vi "AMview.vi"() -> ()   [LabVIEW 2014]
uses:
  TypeDefs/Color.ctl
  TypeDefs/SCAN.ctl
  TypeDefs/Poly2DwSlope.ctl
  TypeDefs/Point2DwSlope.ctl
  TypeDefs/CameraEvent.ctl
  TypeDefs/Camera.ctl
  <vilib>/Utility/miscctls.llb/LV3DPointTypeDef.ctl
  <vilib>/Utility/miscctls.llb/LVStringsAndValuesArrayTypeDef_U16.ctl
  TypeDefs/Point3D.ctl
  <vilib>/picture/3D Picture Control/Object/Add Object (no reference).vi
  <vilib>/picture/3D Picture Control/Object/Create Object (name).vi
  <vilib>/xml/Close Reference(Node).vi
  <vilib>/picture/3D Picture Control/NI_3D Picture Control.lvlib
  <vilib>/xml/NI_XML.lvlib
  <resource>/objmgr/DOMUserDefRef.rc
panel:
  out "SCAN":T1
  in  "stop":bool
  in  "Toolbar":T4(tab)
  in  "Load":bool
  in  "Line Width":dbl=1.0
  in  "Color Off":T5={"Alpha"=1.0, "Color"=0} {"Alpha" min=0.0 max=1.0 scale=0.0..1.0}
  in  "Line Color":u32(colorbox)=6618880
  in  "Reset":bool
  in  "Ports":enum16{"One Viewport", "Four Viewports"}(ring)
  in  "Build Plate Color":u32(colorbox)=6618880
  in  "Color On":T5={"Alpha"=1.0, "Color"=0} {"Alpha" min=0.0 max=1.0 scale=0.0..1.0}
  in  "Scale":bool
  in  "Percent":dbl=50.0 min=1.0 max=200.0
  in  "ZT":dbl=1.0
  in  "ZPT":bool
  in  "ZNT":bool
  in  "YT":dbl=1.0
  in  "YPT":bool
  in  "YNT":bool
  in  "XT":dbl=1.0
  in  "XPT":bool
  in  "XNT":bool
  in  "Zcen":dbl
  in  "Ycen":dbl
  in  "Xcen":dbl
  in  "Zmax":dbl
  in  "Zmin":dbl
  in  "Ymax":dbl
  in  "Ymin":dbl
  in  "Xmax":dbl
  in  "Xmin":dbl
  in  "ZR":dbl=90.0
  in  "ZRR":bool
  in  "ZLR":bool
  in  "YR":dbl=90.0
  in  "YRR":bool
  in  "YLR":bool
  in  "XR":dbl=90.0
  in  "XRR":bool
  in  "XLR":bool
  in  "Model Selector":u16(ring) items=["GE_SnapBlock_18x9_Repaired"]
  in  "Model Color":T5={"Alpha"=1.0, "Color"=0} {"Alpha" min=0.0 max=1.0 scale=0.0..1.0}
  in  "Layer Thickness":dbl=1.0
  in  "Beam Size":dbl=1.0
  in  "Build Size":dbl=100.0
  in  "SavePath":bool
  in  "Slice":bool
  in  "Z":dbl
  in  "SaveSCAN":bool
  in  "SaveXML":bool
  in  "GenLayer":bool
  out "XML":string
  # "X-->"
  # "Translation"
  # "Scale/Sym"
  # "Rotation"
  # "Bounds"
  # "Y-->"
  # "Z-->"
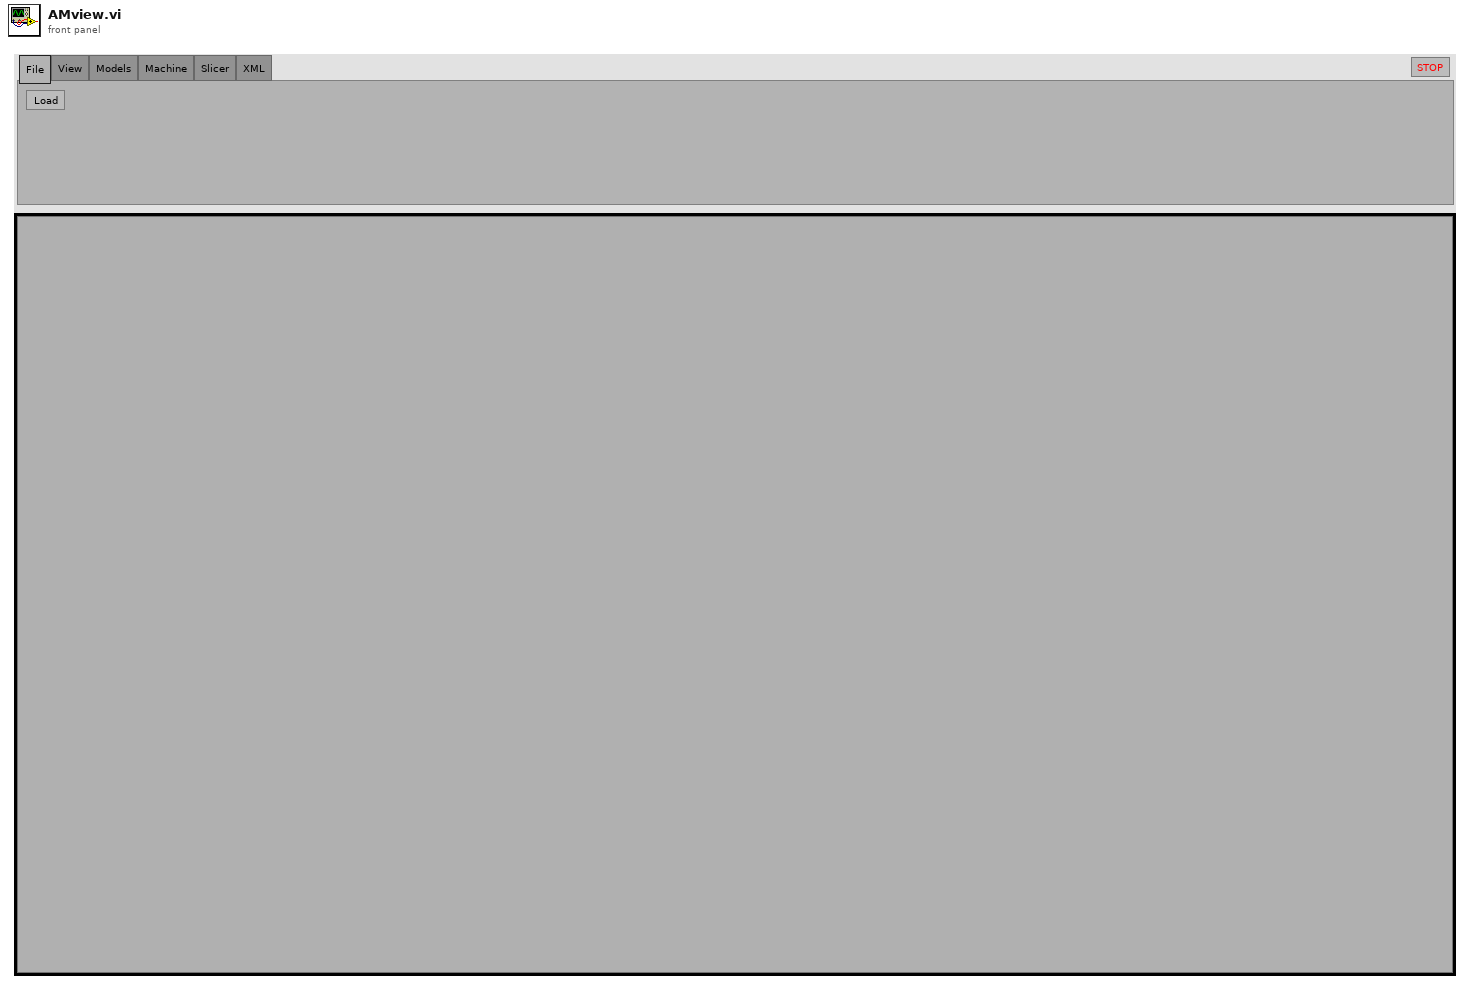
[diagram p1: front panel]
types:
  T1 = typedef "SCAN.ctl" = cluster{"Polys":T2[], "Path":cluster{"VertexArray":T3[], "OnOffAr":enum16{"On", "Off"}[]}}
  T2 = typedef "Poly2DwSlope.ctl" = cluster{"VertexArray":T3[]}
  T3 = typedef "Point2DwSlope.ctl" = cluster{"X":sgl, "Y":sgl, "Slope":dbl}
  T4 = enum32{"File", "View", "Models", "Machine", "Slicer", "XML"}
  T5 = typedef "Color.ctl" = cluster{"Alpha":dbl, "Color":u32}
  T6 = enum16{"Add", "Get", "Scale", "Rotate", "Translate", "Symmetry", "Clear"}
  T7 = enum16{"New", "Find", "FindPattern", "GetTable", "Clear"}
  T8 = typedef "LVStringsAndValuesArrayTypeDef_U16.ctl" = cluster{"String":string, "Value":u16}[]
  T9 = typedef "CameraEvent.ctl" = cluster{"Camera":T10, "Task":enum16{"redraw", "setTo", "setToUpdate"}}
  T10 = typedef "Camera.ctl" = cluster{"Camera Position":T11, "Target":T11, "Up Direction":T11}
  T11 = typedef "LV3DPointTypeDef.ctl" = cluster{"X":sgl, "Y":sgl, "Z":sgl}
  T12 = enum16{"Add", "Get", "Scale", "Rotate", "Translate", "Symmetry"}
  T13 = enum16{"Overall", "Per Primitive", "Per Vertex", "Binding Off"}
  T14 = enum16{"Points", "Lines", "Line Strip", "Line Loop", "Triangles", "Triangle Strip", "Triangle Fan", "Quads", "Quad Strip", "Polygon"}
  T15 = cluster{"Axis":enum16{"X", "Y", "Z"}, "Angle":sgl}
  T16 = typedef "Point3D.ctl" = cluster{"X":sgl, "Y":sgl, "Z":sgl}
  T17 = typedef "TriangleFace.ctl" = cluster{"Normal":T16, "Vertex1":T16, "Vertex2":T16, "Vertex3":T16}
  T18 = typedef "Line2D.ctl" = cluster{"Vertex1":T3, "Vertex2":T3, "Slope":dbl}
  T19 = cluster{"VertexArray":T3[], "OnOffAr":enum16{"On", "Off"}[]}
  T20 = cluster{"Polys":T2[], "Path":cluster{"VertexArray":T3[], "OnOffAr":enum16{"On", "Off"}[]}}
  T21 = cluster{"VertexArray":T3[], enum16{"On", "Off"}[]}
  T22 = cluster{"VertexArray":T3[], "OnOffAr":enum16{"On", "Off"}[]}[]
  T23 = typedef "XYonOffArray.ctl" = cluster{"X":dbl, "Y":dbl, "OnOff":bool}[]
  T24 = typedef "LVRGBAColorTypeDef.ctl" = cluster{"Red":sgl, "Green":sgl, "Blue":sgl, "Alpha":sgl}
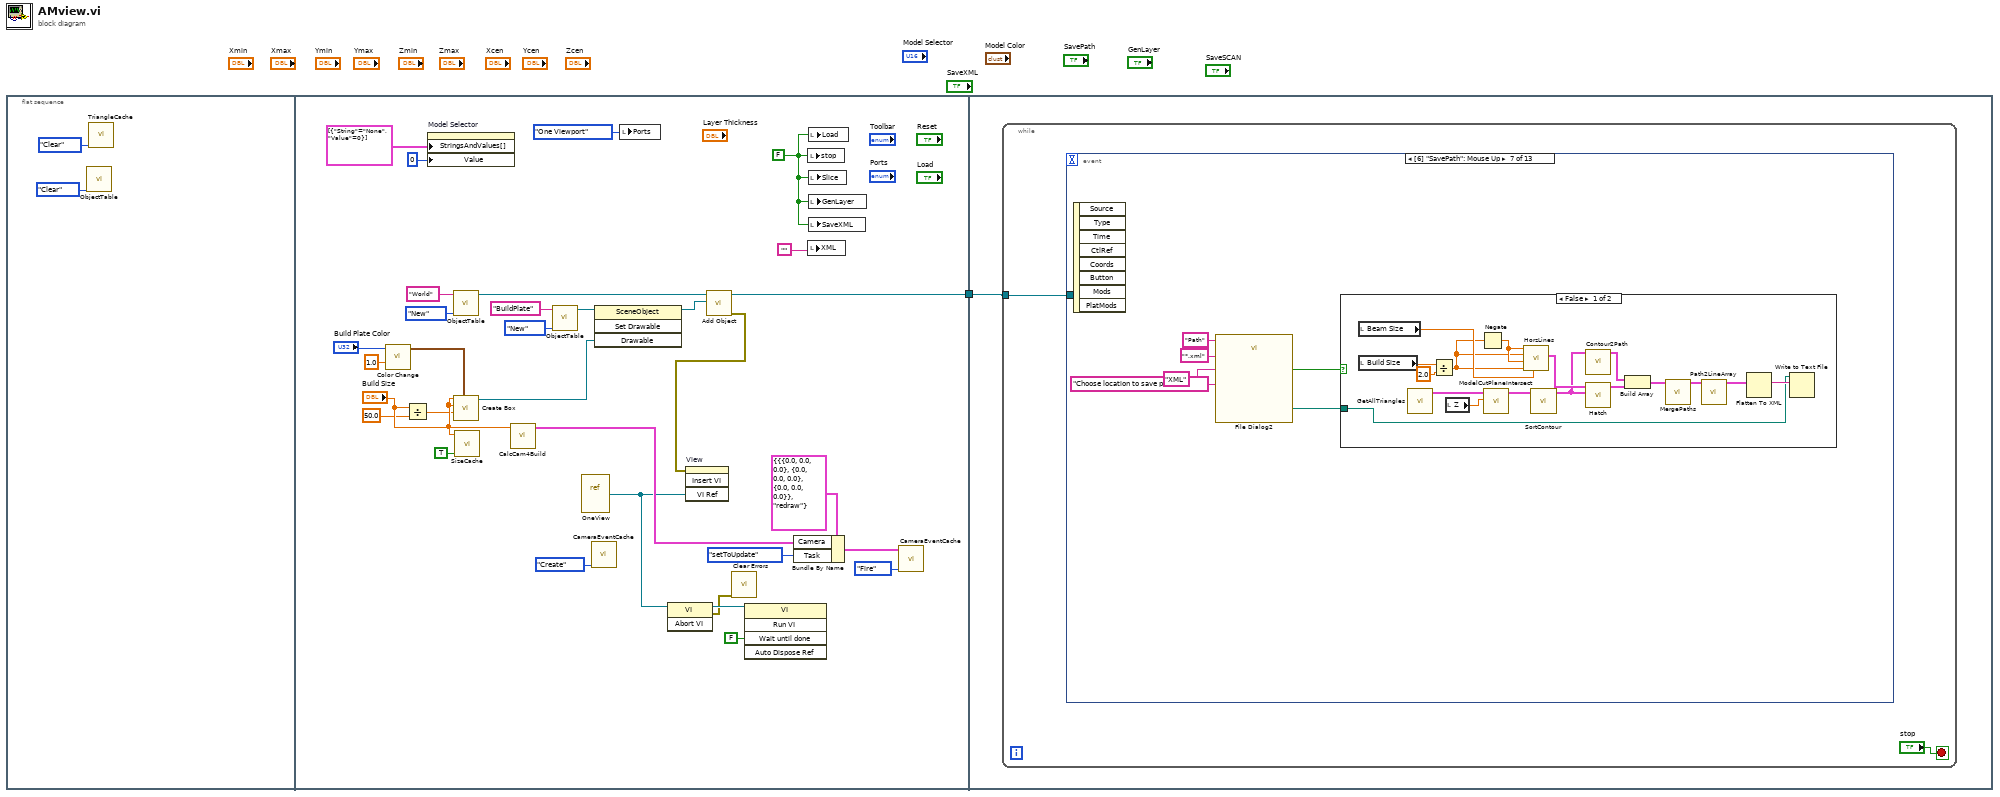
[diagram p0: block diagram]
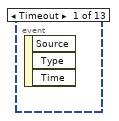
[diagram p2: hidden frame]
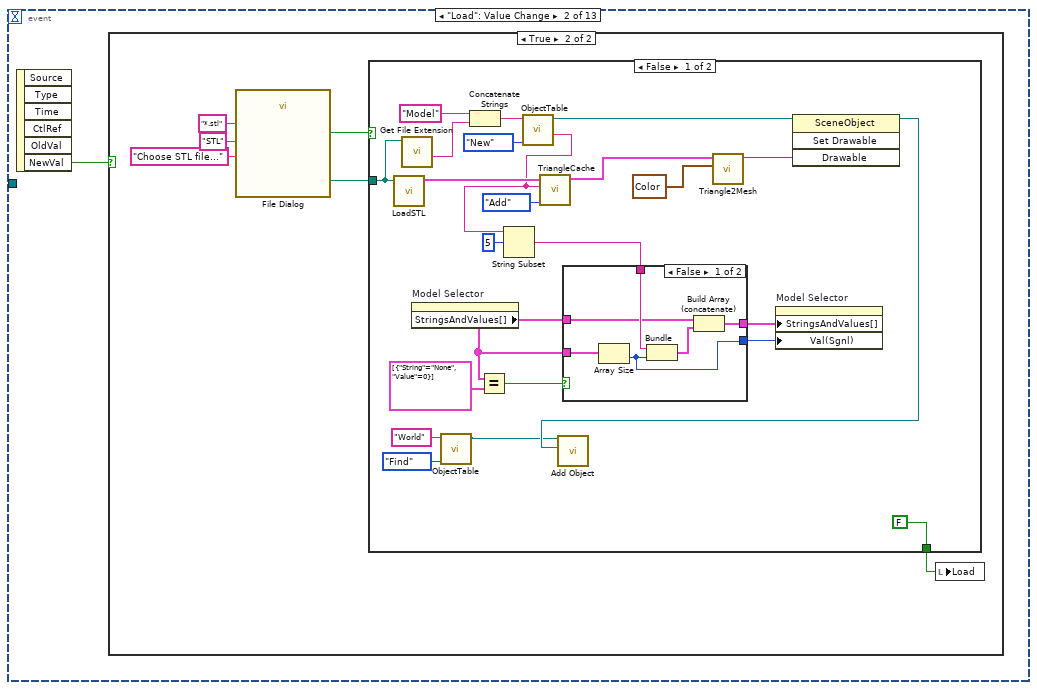
[diagram p3: hidden frame]
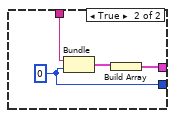
[diagram p5: hidden frame]
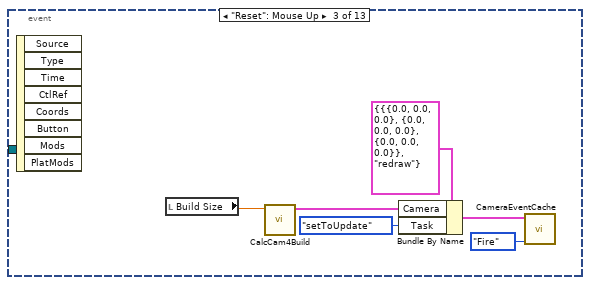
[diagram p7: hidden frame]
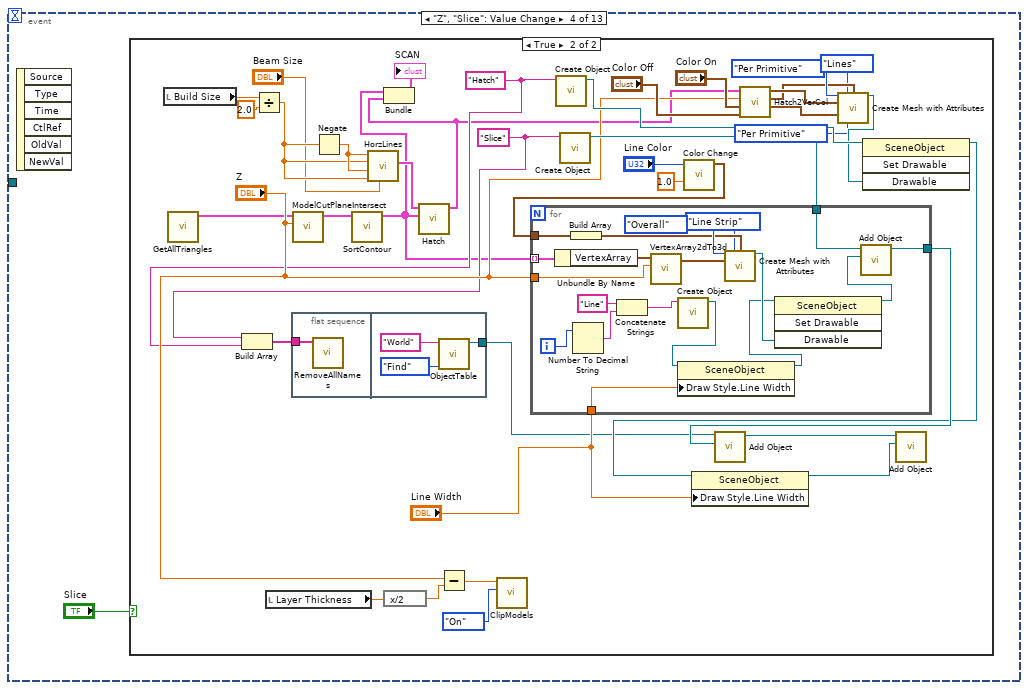
[diagram p8: hidden frame]
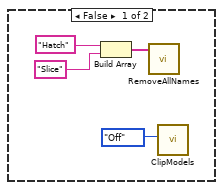
[diagram p9: hidden frame]
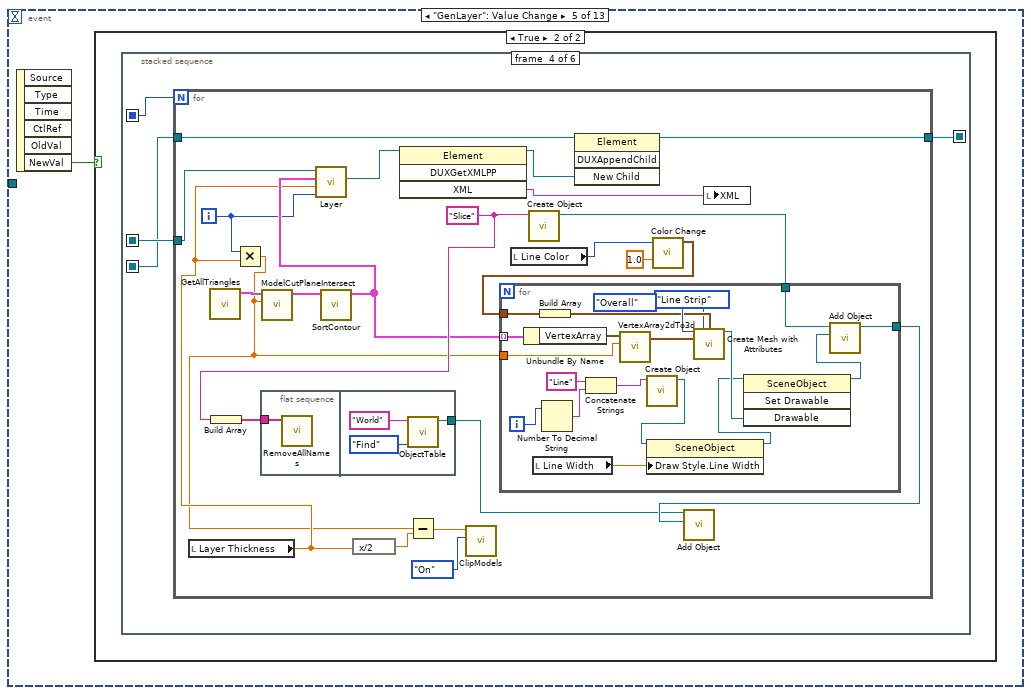
[diagram p10: hidden frame]
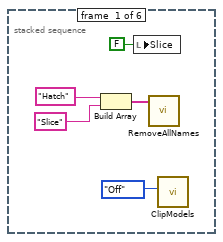
[diagram p12: hidden frame]
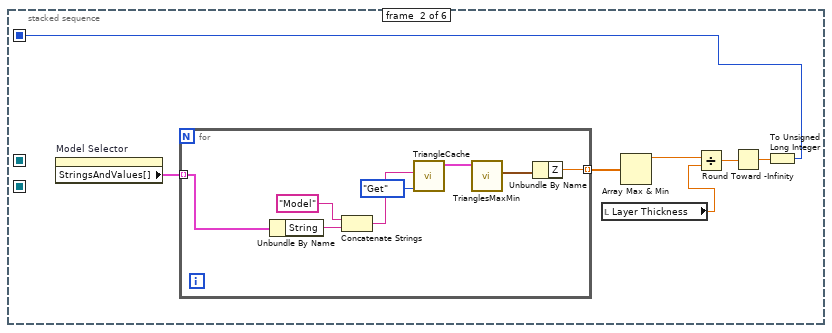
[diagram p13: hidden frame]
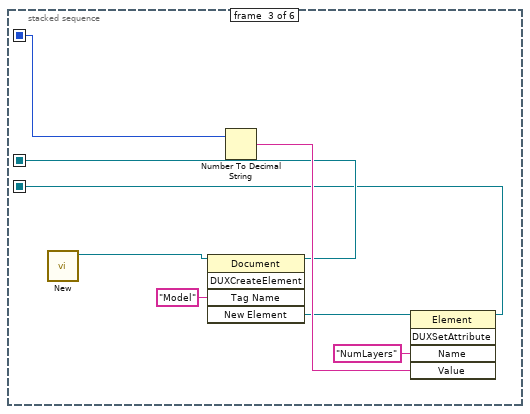
[diagram p14: hidden frame]
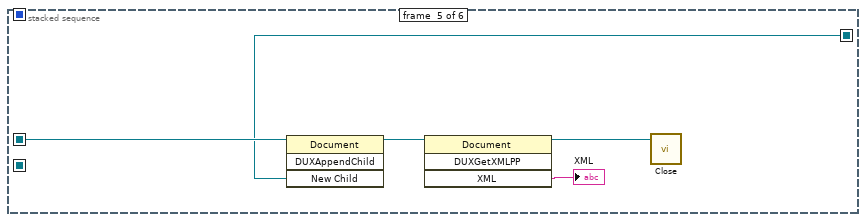
[diagram p15: hidden frame]
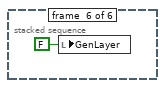
[diagram p16: hidden frame]
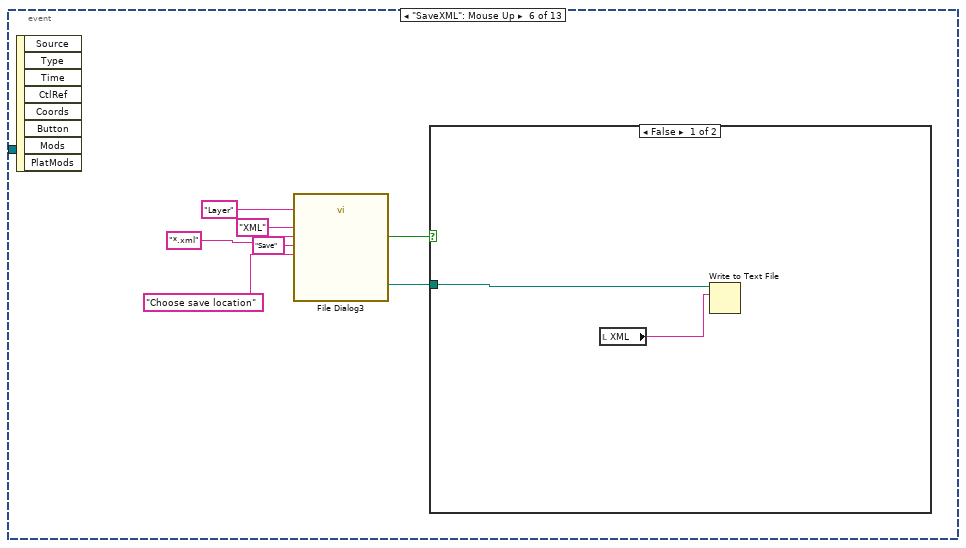
[diagram p17: hidden frame]
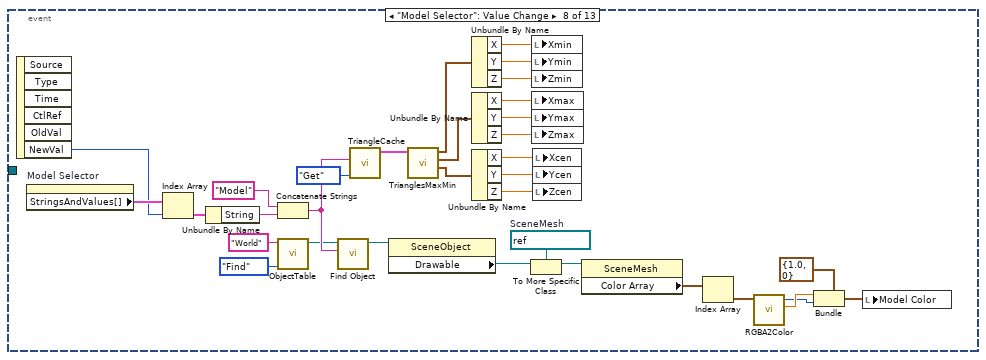
[diagram p20: hidden frame]
diagram:
  n1 = flat-sequence {
    tunnel: [w13] -> w1
    tunnel: w1 -> [w36]
    frame #0 {
      n2 = call "ObjectTable.vi"("ObjectStoreSelector"=T7."Clear") -> ()  [unwired: 6 in, 5 out]
      n3 = call "TriangleCache.vi"("TriangleOperations"=T6."Clear") -> ()  [unwired: 10 in, 1 out]
    }
    frame #1 {
      w5 = FALSE ("stop")
      n4 = call <vilib>:"Color Change.vi"("Alpha"=1.0, "Color"="Build Plate Color") -> ("RGBA"=w17:cluster{"R":sgl, "G":sgl, "B":sgl, "A":sgl})  [unwired: 9 in]
      n5 = Divide(x="Build Size", y=50.0) -> (x/y=w15:dbl)
      n6 = property on="Model Selector" class="Ring (strict)"("StringsAndValues[]"=T8 [{"String"="None", "Value"=0}] ("Strings And Values []"), "Value"=0) -> ()  [unwired: 2 in, 2 out]
      n7 = call "ObjectTable.vi"("ObjectStoreSelector"=enum16{"New", "Find", "FindPattern", "GetTable"}."New", "Name"="World") -> ("ObjectRef"=w31:refnum<vi>)  [unwired: 5 in, 4 out]
      n8 = call <vilib>:"Create Box.vi"("Color"=w17, "Length Z"=w15, "Length Y"="Build Size", "Length X"="Build Size") -> ("New Box Refnum"=w19:refnum<vi>)  [unwired: 6 in, 1 out]
      n9 = call "SizeCache.vi"("Set"=TRUE, "SizeIn"="Build Size") -> ()  [unwired: 9 in, 1 out]
      n10 = call "CalcCam4Build.vi"("BuildSize"="Build Size") -> ("CamOut"=w25:T10)  [unwired: 10 in]
      n11 = call "ObjectTable.vi"("ObjectStoreSelector"=enum16{"New", "Find", "FindPattern", "GetTable"}."New", "Name"="BuildPlate") -> ("ObjectRef"=w33:refnum<vi>)  [unwired: 5 in, 4 out]
      n12 = vi-ref "OneView.vi"() -> (w9:refnum<vi>)
      n13 = call "CameraEventCache.vi"("Operation"=enum16{"Create", "GetRef", "Fire"}."Create") -> ()  [unwired: 10 in, 1 out]
      n14 = invoke class="SceneObject" method="Set Drawable"(reference=w33, "Drawable"=w19) -> (reference out=w20:refnum<vi>)  [unwired: 2 in, 3 out]
      n15 = local write "Ports"(enum16{"One Viewport", "Four Viewports"}."One Viewport" ("Ports")) -> ()
      n16 = invoke class="VI" method="Abort VI"(reference=w9) -> (reference out=w10:refnum<vi>, error out=w6:errorcluster)  [unwired: 2 in, 1 out]
      n17 = call-poly <vilib>:"Add Object.vi"("New Object In"=w20, "Scene Object In"=w31) -> ("error out"=w35:errorcluster, "Scene Object Out"=w13:refnum<vi>)  [unwired: 8 in]
      n18 = invoke on="View" class="SubPanel" method="Insert VI"(error in=w35, "VI Ref"=w9) -> ()  [unwired: 2 in, 4 out]
      n19 = call <vilib>:"Clear Errors.vi"("error in (no error)"=w6) -> ()  [unwired: 5 in, 2 out]
      n20 = invoke class="VI" method="Run VI"(reference=w10, "Wait until done"=FALSE ("Wait Until Done")) -> ()  [unwired: 3 in, 5 out]
      n21 = Bundle By Name(cluster=T9 {"Camera"={"Camera Position"={"X"=0.0, "Y"=0.0, "Z"=0.0}, "Target"={"X"=0.0, "Y"=0.0, "Z"=0.0}, "Up Direction"={"X"=0.0, "Y"=0.0, "Z"=0.0}}, "Task"=enum."redraw"} ("CameraEvent"), "Camera"=w25, "Task"=enum16{"redraw", "setTo", "setToUpdate"}."setToUpdate") -> (w24:T9)
      n22 = local write "stop"(w5) -> ()
      n23 = local write "XML"("") -> ()
      n24 = local write "Load"(w5) -> ()
      n25 = local write "Slice"(w5) -> ()
      n26 = local write "GenLayer"(w5) -> ()
      n27 = local write "SaveXML"(w5) -> ()
      n28 = call "CameraEventCache.vi"("Operation"=enum16{"Create", "GetRef", "Fire"}."Fire", "CameraEvent"=w24) -> ()  [unwired: 9 in, 1 out]
    }
    frame #2 {
      n29 = while {
        tunnel: w36 -> [w37]
        stop <- "stop" stop-if-true
        n30 = event shown="[6] \"SavePath\": Mouse Up" {
          selector: _ -> [_ _ _ _ _ _ _ _ _ _ _ _ _]
          dyn-events: _ -> [_ _ _ _ _ _ _ _ _ _ _ _ _]
          timeout: _ -> [_ _ _ _ _ _ _ _ _ _ _ _ _]
          tunnel: w37 -> [_ _ _ _ _ _ _ _ _ _ _ _ _]
          event Timeout {
            n31 = event-data() -> ()  [unwired: 1 in, 3 out]
          }
          event "Load": Value Change {
            n32 = event-data() -> ("NewVal"=w39:bool)  [unwired: 1 in, 5 out]
            n33 = case shown="True" w39 {
              frame False {
              }
              frame True {
                n34 = call "File Dialog"("prompt"="Choose STL file...", "pattern (all files)"="*.stl", "pattern label"="STL") -> ("selected path"=w41:path, "cancelled"=w42:bool)  [unwired: 9 in, 2 out]
                n35 = case shown="False" w42 {
                  tunnel: w41 -> [w54 _]
                  tunnel: [FALSE _] -> w40
                  frame False {
                    n36 = call "LoadSTL.vi"("STL Path"=w54) -> ("Triangles"=w59:T17[])  [unwired: 8 in, 2 out]
                    n37 = call <vilib>:"Get File Extension.vi"("file"=w54) -> ("filename without extension"=w53:string)  [unwired: 7 in, 3 out]
                    n38 = property on="Model Selector" class="Ring (strict)"() -> ("StringsAndValues[]"=w48:T8)  [unwired: 2 in, 2 out]
                    n39 = call "ObjectTable.vi"("ObjectStoreSelector"=enum16{"New", "Find", "FindPattern", "GetTable"}."Find", "Name"="World") -> ("ObjectRef"=w63:refnum<vi>)  [unwired: 5 in, 4 out]
                    n40 = Concatenate Strings("Model" ("Name"), w53) -> (w66:string)
                    n41 = Equal?(x=w48, y=T8 [{"String"="None", "Value"=0}] ("Strings And Values []")) -> (x = y?=w47:bool)
                    n42 = call "ObjectTable.vi"("ObjectStoreSelector"=enum16{"New", "Find", "FindPattern", "GetTable"}."New", "Name"=w66) -> ("UniqueName"=w51:string, "ObjectRef"=w64:refnum<vi>)  [unwired: 5 in, 3 out]
                    n43 = String Subset(string=w51, offset (0)=5) -> (substring=w52:string)  [unwired: 1 in]
                    n44 = call "TriangleCache.vi"("TriangleOperations"=T12."Add", "ModelName"=w51, "TrianglesIn"=w59) -> ("TrianglesOut"=w58:T17[])  [unwired: 8 in]
                    n45 = case shown="False" w47 {
                      tunnel: [w74 w77] -> w56
                      tunnel: [w73 w76] -> w55
                      tunnel: w52 -> [w72 w79]
                      tunnel: w48 -> [w71 _]
                      tunnel: w48 -> [w70 _]
                      frame False {
                        n46 = Array Size(array=w70) -> (size(s)=w73:i32)
                        n47 = Bundle("UniqueName"=w72, w73) -> (w75:cluster{"UniqueName":string, i32})  [unwired: 1 in]
                        n48 = Build Array (concatenate)(w71, w75) -> (w74:cluster{"UniqueName":string, "Value":i32}[])
                      }
                      frame True {
                        w76 = 0
                        n49 = Bundle("UniqueName"=w79, w76) -> (w78:cluster{"UniqueName":string, i32})  [unwired: 1 in]
                        n50 = Build Array(w78) -> (w77:cluster{"UniqueName":string, i32}[])
                      }
                    }
                    n51 = call "Triangle2Mesh.vi"("Color"=T5 {"Alpha"=1.0, "Color"=16711680}, "Triangles"=w58) -> ("Refnum"=w60:refnum<vi>)  [unwired: 9 in]
                    n52 = property on="Model Selector" class="Ring (strict)"("StringsAndValues[]"=w56, "Val(Sgnl)"=w55) -> ()  [unwired: 2 in, 2 out]
                    n53 = invoke class="SceneObject" method="Set Drawable"(reference=w64, "Drawable"=w60) -> (reference out=w69:refnum<vi>)  [unwired: 2 in, 3 out]
                    n54 = call-poly <vilib>:"Add Object.vi"("New Object In"=w69, "Scene Object In"=w63) -> ()  [unwired: 8 in, 2 out]
                  }
                  frame True {
                  }
                }
                n55 = local write "Load"(w40) -> ()
              }
            }
          }
          event "Reset": Mouse Up {
            n56 = event-data() -> ()  [unwired: 1 in, 8 out]
            n57 = local read "Build Size"() -> (w82:dbl)
            n58 = call "CalcCam4Build.vi"("BuildSize"=w82) -> ("CamOut"=w83:T10)  [unwired: 10 in]
            n59 = Bundle By Name(cluster=T9 {"Camera"={"Camera Position"={"X"=0.0, "Y"=0.0, "Z"=0.0}, "Target"={"X"=0.0, "Y"=0.0, "Z"=0.0}, "Up Direction"={"X"=0.0, "Y"=0.0, "Z"=0.0}}, "Task"=enum."redraw"} ("CameraEvent"), "Camera"=w83, "Task"=enum16{"redraw", "setTo", "setToUpdate"}."setToUpdate") -> (w81:T9)
            n60 = call "CameraEventCache.vi"("Operation"=enum16{"Create", "GetRef", "Fire"}."Fire", "CameraEvent"=w81) -> ()  [unwired: 9 in, 1 out]
          }
          event "Z", "Slice": Value Change {
            n61 = event-data() -> ()  [unwired: 1 in, 6 out]
            n62 = case shown="True" "Slice" {
              frame False {
                n63 = Build Array("Hatch", "Slice") -> (w89:string[])
                n64 = call "RemoveAllNames.vi"("Names"=w89) -> ()  [unwired: 11 in]
                n65 = call "ClipModels.vi"("Clip Plane State"=enum16{"Inherit Value", "Off", "On"}."Off") -> ()  [unwired: 11 in]
              }
              frame True {
                w96 = "Hatch" ("Name")
                w97 = "Slice" ("Name")
                n66 = local read "Build Size"() -> (w127:dbl)
                n67 = call "GetAllTriangles.vi"() -> ("AllTriangles"=w100:T17[])  [unwired: 11 in]
                n68 = Build Array(w97, w96) -> (w95:string[])
                n69 = Divide(x=w127, y=2.0) -> (x/y=w124:dbl)
                n70 = local read "Layer Thickness"() -> (w102:dbl)
                n71 = flat-sequence {
                  tunnel: w95 -> [w130]
                  tunnel: [w131] -> w94
                  frame #0 {
                    n72 = call "RemoveAllNames.vi"("Names"=w130) -> ()  [unwired: 11 in]
                  }
                  frame #1 {
                    n73 = call "ObjectTable.vi"("ObjectStoreSelector"=T7."Find", "Name"="World") -> ("ObjectRef"=w131:refnum<vi>)  [unwired: 5 in, 4 out]
                  }
                }
                n74 = call "ModelCutPlaneIntersect.vi"("CuttingZ"="Z", "Triangles"=w100) -> ("LineArray"=w129:T18[])  [unwired: 8 in, 1 out]
                n75 = Negate(x=w124) -> (-x=w125:dbl)
                n76 = call "SortContour.vi"("LineArray"=w129) -> ("Polys"=w93:T2[])  [unwired: 10 in]
                n77 = call "HorzLines.vi"("Spacing"="Beam Size", "yMax"=w124, "yMin"=w125, "xMax"=w124, "xMin"=w125) -> ("Poly2D"=w128:T2)  [unwired: 5 in, 1 out]
                n78 = expression code="x/2"(w102) -> (w101:dbl)
                n79 = call "Hatch.vi"("Polys"=w93, "Hatch"=w128) -> ("Path"=w92:T19)  [unwired: 9 in]
                n80 = Bundle("Polys"=w93, "Path"=w92) -> (→"SCAN":T20)  [unwired: 1 in]
                n81 = Subtract(x="Z", y=w101) -> (x-y=w99:dbl)
                n82 = call "ClipModels.vi"("Clip Plane State"=enum16{"Inherit Value", "Off", "On"}."On", "Z"=w99) -> ()  [unwired: 10 in]
                n83 = call-poly <vilib>:"Create Object.vi"("Name"=w96) -> ("Scene:New Object"=w112:refnum<vi>)  [unwired: 9 in, 1 out]
                n84 = call-poly <vilib>:"Create Object.vi"("Name"=w97) -> ("Scene:New Object"=w121:refnum<vi>)  [unwired: 9 in, 1 out]
                n85 = call <vilib>:"Color Change.vi"("Alpha"=1.0, "Color"="Line Color") -> ("RGBA"=w122:cluster{"R":sgl, "G":sgl, "B":sgl, "A":sgl})  [unwired: 9 in]
                n86 = for {
                  tunnel: w93 -> [w151] mode=indexing
                  tunnel: "Z" -> [w149]
                  tunnel: w122 -> [w147]
                  tunnel: w121 -> [w140]
                  tunnel: [w139] -> w120
                  tunnel: "Line Width" -> [w134]
                  i -> [w143]
                  n87 = Unbundle By Name(w151) -> ("VertexArray"=w150:T3[])
                  n88 = Build Array(w147) -> (w146:cluster{"R":sgl, "G":sgl, "B":sgl, "A":sgl}[])
                  n89 = Number To Decimal String(number=w143) -> (decimal integer string=w142:string)  [unwired: 1 in]
                  n90 = Concatenate Strings("Line" ("string"), w142) -> (w141:string)
                  n91 = call "VertexArray2dTo3d.vi"("Z"=w149, "VertexArray2D"=w150) -> ("VertexArray3D"=w148:T16[])  [unwired: 9 in]
                  n92 = call-poly <vilib>:"Create Object.vi"("Name"=w141) -> ("Scene:New Object"=w136:refnum<vi>)  [unwired: 9 in, 1 out]
                  n93 = property class="SceneObject"(reference=w136, "Draw Style.Line Width"=w134) -> (reference out=w135:refnum<vi>)  [unwired: 1 in, 1 out]
                  n94 = call <vilib>:"Create Mesh with Attributes.vi"("Draw Mode"=T14."Line Strip", "Color Binding Mode"=T13."Overall", "Color Array"=w146, "Vertex Array"=w148) -> ("New Mesh Refnum"=w138:refnum<vi>)  [unwired: 10 in, 1 out]
                  n95 = invoke class="SceneObject" method="Set Drawable"(reference=w135, "Drawable"=w138) -> (reference out=w137:refnum<vi>)  [unwired: 2 in, 3 out]
                  n96 = call-poly <vilib>:"Add Object.vi"("New Object In"=w137, "Scene Object In"=w140) -> ("Scene Object Out"=w139:refnum<vi>)  [unwired: 8 in, 1 out]
                }
                n97 = call-poly <vilib>:"Add Object.vi"("New Object In"=w120, "Scene Object In"=w94) -> ("Scene Object Out"=w110:refnum<vi>)  [unwired: 8 in, 1 out]
                n98 = call "Hatch2VerCol.vi"("Color Off"="Color Off", "Color On"="Color On", "Z"="Z", "Path"=w92) -> ("Normals"=w105:T16[], "Colors"=w114:cluster{"R":sgl, "G":sgl, "B":sgl, "A":sgl}[], "VertexArray3d"=w115:T16[])  [unwired: 5 in]
                n99 = call <vilib>:"Create Mesh with Attributes.vi"("Draw Mode"=T14."Lines", "Color Binding Mode"=T13."Per Primitive", "Color Array"=w114, "Vertex Array"=w115, "Normal Array"=w105, "Normal Binding Mode"=T13."Per Primitive") -> ("New Mesh Refnum"=w111:refnum<vi>)  [unwired: 8 in, 1 out]
                n100 = invoke class="SceneObject" method="Set Drawable"(reference=w112, "Drawable"=w111) -> (reference out=w108:refnum<vi>)  [unwired: 2 in, 3 out]
                n101 = property class="SceneObject"(reference=w108, "Draw Style.Line Width"="Line Width") -> (reference out=w106:refnum<vi>)  [unwired: 1 in, 1 out]
                n102 = call-poly <vilib>:"Add Object.vi"("New Object In"=w106, "Scene Object In"=w110) -> ()  [unwired: 8 in, 2 out]
              }
            }
          }
          event "GenLayer": Value Change {
            n103 = event-data() -> ("NewVal"=w153:bool)  [unwired: 1 in, 5 out]
            n104 = case shown="True" w153 {
              frame False {
              }
              frame True {
                n105 = stacked-sequence {
                  seq-local: [_ w159 _ _ _ _] -> [_ _ w176 w185 _ _]
                  seq-local: [_ _ w175 _ _ _] -> [_ _ _ w184 w236 _]
                  seq-local: [_ _ w174 _ _ _] -> [_ _ _ w183 _ _]
                  seq-local: [_ _ _ w182 _ _] -> [_ _ _ _ w235 _]
                  frame #0 {
                    n106 = Build Array("Hatch", "Slice") -> (w156:string[])
                    n107 = local write "Slice"(FALSE ("Slice")) -> ()
                    n108 = call "RemoveAllNames.vi"("Names"=w156) -> ()  [unwired: 11 in]
                    n109 = call "ClipModels.vi"("Clip Plane State"=enum16{"Inherit Value", "Off", "On"}."Off") -> ()  [unwired: 11 in]
                  }
                  frame #1 {
                    n110 = property on="Model Selector" class="Ring (strict)"() -> ("StringsAndValues[]"=w165:T8)  [unwired: 2 in, 2 out]
                    n111 = for {
                      tunnel: w165 -> [w168] mode=indexing
                      tunnel: [w166] -> w164 mode=indexing
                      n112 = Unbundle By Name(w168) -> ("String"=w173:string)
                      n113 = Concatenate Strings("Model" ("string"), w173) -> (w169:string)
                      n114 = call "TriangleCache.vi"("TriangleOperations"=T6."Get", "ModelName"=w169) -> ("TrianglesOut"=w170:T17[])  [unwired: 9 in]
                      n115 = call "TrianglesMaxMin.vi"("Triangles"=w170) -> ("MaxDims"=w167:T16)  [unwired: 8 in, 2 out]
                      n116 = Unbundle By Name(w167) -> ("Z"=w166:sgl)
                    }
                    n117 = local read "Layer Thickness"() -> (w162:dbl)
                    n118 = Array Max & Min(array=w164) -> (max value=w163:sgl)  [unwired: 3 out]
                    n119 = Divide(x=w163, y=w162) -> (x/y=w161:dbl)
                    n120 = Round Toward -Infinity(1:w161) -> (0:w160:dbl)
                    n121 = To Unsigned Long Integer(number=w160) -> (unsigned 32bit integer=w159:u32)
                  }
                  frame #2 {
                    n122 = call <vilib>:"New.vi"() -> ("DOM document out"=w178:refnum<k20>)  [unwired: 8 in, 1 out]
                    n123 = invoke class="Document" method="DUXCreateElement"(reference=w178, "Tag Name"="Model") -> (reference out=w175:refnum<k20>, "New Element"=w177:refnum<k20>)  [unwired: 3 in, 3 out]
                    n124 = Number To Decimal String(number=w176) -> (decimal integer string=w179:string)  [unwired: 1 in]
                    n125 = invoke class="Element" method="DUXSetAttribute"(reference=w177, "Name"="NumLayers", "Value"=w179) -> (reference out=w174:refnum<k20>)  [unwired: 2 in, 4 out]
                  }
                  frame #3 {
                    n126 = for {
                      N: w185 -> [_]
                      tunnel: w184 -> [w195]
                      tunnel: w183 -> [w193]
                      tunnel: [w192] -> w182
                      i -> [w191]
                      w198 = "Slice" ("Name")
                      n127 = local read "Layer Thickness"() -> (w190:dbl)
                      n128 = call "GetAllTriangles.vi"() -> ("AllTriangles"=w201:T17[])  [unwired: 11 in]
                      n129 = Build Array(w198) -> (w197:string[])
                      n130 = Multiply(x=w191, y=w190) -> (x*y=w189:dbl)
                      n131 = flat-sequence {
                        tunnel: w197 -> [w209]
                        tunnel: [w210] -> w196
                        frame #0 {
                          n132 = call "RemoveAllNames.vi"("Names"=w209) -> ()  [unwired: 11 in]
                        }
                        frame #1 {
                          n133 = call "ObjectTable.vi"("ObjectStoreSelector"=T7."Find", "Name"="World") -> ("ObjectRef"=w210:refnum<vi>)  [unwired: 5 in, 4 out]
                        }
                      }
                      n134 = call "ModelCutPlaneIntersect.vi"("CuttingZ"=w189, "Triangles"=w201) -> ("LineArray"=w207:T18[])  [unwired: 8 in, 1 out]
                      n135 = call "SortContour.vi"("LineArray"=w207) -> ("Polys"=w194:T2[])  [unwired: 10 in]
                      n136 = call "Layer.vi"("Index"=w191, "Thickness"=w190, "Contours"=w194, "DocIn"=w195) -> ("Layer"=w188:refnum<k20>)  [unwired: 6 in, 1 out]
                      n137 = expression code="x/2"(w190) -> (w202:dbl)
                      n138 = invoke class="Element" method="DUXGetXMLPP"(reference=w188) -> (reference out=w187:refnum<k20>, "XML"=w186:string)  [unwired: 3 in, 2 out]
                      n139 = Subtract(x=w189, y=w202) -> (x-y=w200:dbl)
                      n140 = call "ClipModels.vi"("Clip Plane State"=enum16{"Inherit Value", "Off", "On"}."On", "Z"=w200) -> ()  [unwired: 10 in]
                      n141 = local read "Line Color"() -> (w208:u32)
                      n142 = call-poly <vilib>:"Create Object.vi"("Name"=w198) -> ("Scene:New Object"=w205:refnum<vi>)  [unwired: 9 in, 1 out]
                      n143 = invoke class="Element" method="DUXAppendChild"(reference=w193, "New Child"=w187) -> (reference out=w192:refnum<k20>)  [unwired: 2 in, 3 out]
                      n144 = call <vilib>:"Color Change.vi"("Alpha"=1.0, "Color"=w208) -> ("RGBA"=w206:cluster{"R":sgl, "G":sgl, "B":sgl, "A":sgl})  [unwired: 9 in]
                      n145 = for {
                        tunnel: w194 -> [w230] mode=indexing
                        tunnel: w189 -> [w228]
                        tunnel: w206 -> [w226]
                        tunnel: w205 -> [w219]
                        tunnel: [w218] -> w204
                        i -> [w222]
                        n146 = Unbundle By Name(w230) -> ("VertexArray"=w229:T3[])
                        n147 = local read "Line Width"() -> (w213:dbl)
                        n148 = Build Array(w226) -> (w225:cluster{"R":sgl, "G":sgl, "B":sgl, "A":sgl}[])
                        n149 = Number To Decimal String(number=w222) -> (decimal integer string=w221:string)  [unwired: 1 in]
                        n150 = Concatenate Strings("Line" ("string"), w221) -> (w220:string)
                        n151 = call "VertexArray2dTo3d.vi"("Z"=w228, "VertexArray2D"=w229) -> ("VertexArray3D"=w227:T16[])  [unwired: 9 in]
                        n152 = call-poly <vilib>:"Create Object.vi"("Name"=w220) -> ("Scene:New Object"=w215:refnum<vi>)  [unwired: 9 in, 1 out]
                        n153 = property class="SceneObject"(reference=w215, "Draw Style.Line Width"=w213) -> (reference out=w214:refnum<vi>)  [unwired: 1 in, 1 out]
                        n154 = call <vilib>:"Create Mesh with Attributes.vi"("Draw Mode"=T14."Line Strip", "Color Binding Mode"=T13."Overall", "Color Array"=w225, "Vertex Array"=w227) -> ("New Mesh Refnum"=w217:refnum<vi>)  [unwired: 10 in, 1 out]
                        n155 = invoke class="SceneObject" method="Set Drawable"(reference=w214, "Drawable"=w217) -> (reference out=w216:refnum<vi>)  [unwired: 2 in, 3 out]
                        n156 = call-poly <vilib>:"Add Object.vi"("New Object In"=w216, "Scene Object In"=w219) -> ("Scene Object Out"=w218:refnum<vi>)  [unwired: 8 in, 1 out]
                      }
                      n157 = call-poly <vilib>:"Add Object.vi"("New Object In"=w204, "Scene Object In"=w196) -> ()  [unwired: 8 in, 2 out]
                      n158 = local write "XML"(w186) -> ()
                    }
                  }
                  frame #4 {
                    n159 = invoke class="Document" method="DUXAppendChild"(reference=w236, "New Child"=w235) -> (reference out=w234:refnum<k20>)  [unwired: 2 in, 3 out]
                    n160 = invoke class="Document" method="DUXGetXMLPP"(reference=w234) -> (reference out=w232:refnum<k20>, "XML"=→"XML":string)  [unwired: 3 in, 2 out]
                    n161 = call-poly <vilib>:"Close.vi"("node"=w232) -> ()  [unwired: 8 in, 1 out]
                  }
                  frame #5 {
                    n162 = local write "GenLayer"(FALSE ("GenLayer")) -> ()
                  }
                }
              }
            }
          }
          event "SaveXML": Mouse Up {
            n163 = event-data() -> ()  [unwired: 1 in, 8 out]
            n164 = call "File Dialog3"("prompt"="Choose save location", "button label"="Save", "default name"="Layer", "pattern (all files)"="XML", "pattern label"="*.xml") -> ("selected path"=w238:path, "cancelled"=w239:bool)  [unwired: 7 in, 2 out]
            n165 = case shown="False" w239 {
              tunnel: w238 -> [w245 _]
              frame False {
                n166 = local read "XML"() -> (w246:string)
                n167 = Write to Text File(file (use dialog)=w245, text=w246) -> ()  [unwired: 2 in, 3 out]
              }
              frame True {
              }
            }
          }
          event "SavePath": Mouse Up {
            n168 = event-data() -> ()  [unwired: 1 in, 8 out]
            n169 = call "File Dialog2"("prompt"="Choose location to save path...", "default name"="Path", "pattern (all files)"="*.xml", "pattern label"="XML") -> ("selected path"=w248:path, "cancelled"=w249:bool)  [unwired: 8 in, 2 out]
            n170 = case shown="False" w249 {
              tunnel: w248 -> [w258 _]
              frame False {
                n171 = local read "Beam Size"() -> (w268:dbl)
                n172 = local read "Build Size"() -> (w265:dbl)
                n173 = call "GetAllTriangles.vi"() -> ("AllTriangles"=w261:T17[])  [unwired: 11 in]
                n174 = Divide(x=w265, y=2.0) -> (x/y=w262:dbl)
                n175 = local read "Z"() -> (w269:dbl)
                n176 = Negate(x=w262) -> (-x=w263:dbl)
                n177 = call "ModelCutPlaneIntersect.vi"("CuttingZ"=w269, "Triangles"=w261) -> ("LineArray"=w267:T18[])  [unwired: 8 in, 1 out]
                n178 = call "HorzLines.vi"("Spacing"=w268, "yMax"=w262, "yMin"=w263, "xMax"=w262, "xMin"=w263) -> ("Poly2D"=w266:T2)  [unwired: 5 in, 1 out]
                n179 = call "SortContour.vi"("LineArray"=w267) -> ("Polys"=w257:T2[])  [unwired: 10 in]
                n180 = call "Contour2Path.vi"("Polys"=w257) -> ("Path"=w255:T21)  [unwired: 10 in]
                n181 = call "Hatch.vi"("Polys"=w257, "Hatch"=w266) -> ("Path"=w256:T19)  [unwired: 9 in]
                n182 = Build Array(w255, w256) -> (w253:T22)
                n183 = call "MergePaths.vi"("PathArray"=w253) -> ("PathOut"=w254:T19)  [unwired: 10 in]
                n184 = call "Path2LineArray.vi"("Path"=w254) -> ("LineArray"=w260:T23)  [unwired: 10 in]
                n185 = Flatten To XML(anything=w260) -> (xml string=w259:string)
                n186 = Write to Text File(file (use dialog)=w258, text=w259) -> ()  [unwired: 2 in, 3 out]
              }
              frame True {
              }
            }
          }
          event "Model Selector": Value Change {
            w297 = refnum<vi> refnum  # SceneMesh
            n187 = event-data() -> ("NewVal"=w301:u16)  [unwired: 1 in, 5 out]
            n188 = property on="Model Selector" class="Ring (strict)"() -> ("StringsAndValues[]"=w302:T8)  [unwired: 2 in, 2 out]
            n189 = Index Array(array=w302, index=w301) -> (element=w300:cluster{"String":string, "Value":u16})
            n190 = Unbundle By Name(w300) -> ("String"=w299:string)
            n191 = Concatenate Strings("Model" ("string"), w299) -> (w274:string)
            n192 = call "ObjectTable.vi"("ObjectStoreSelector"=T7."Find", "Name"="World") -> ("ObjectRef"=w271:refnum<vi>)  [unwired: 5 in, 4 out]
            n193 = call <vilib>:"Find Object.vi"("Object Name"=w274, "Scene Refnum"=w271) -> ("Object Refnum"=w270:refnum<vi>)  [unwired: 8 in, 1 out]
            n194 = call "TriangleCache.vi"("TriangleOperations"=T6."Get", "ModelName"=w274) -> ("TrianglesOut"=w288:T17[])  [unwired: 9 in]
            n195 = property class="SceneObject"(reference=w270) -> ("Drawable"=w275:refnum<vi>)  [unwired: 1 in, 2 out]
            n196 = call "TrianglesMaxMin.vi"("Triangles"=w288) -> ("Center"=w285:T16, "MaxDims"=w286:T16, "MinDims"=w287:T16)  [unwired: 8 in]
            n197 = Unbundle By Name(w287) -> ("X"=w284:sgl, "Y"=w283:sgl, "Z"=w282:sgl)
            n198 = Unbundle By Name(w286) -> ("X"=w281:sgl, "Y"=w280:sgl, "Z"=w279:sgl)
            n199 = Unbundle By Name(w285) -> ("X"=w278:sgl, "Y"=w277:sgl, "Z"=w276:sgl)
            n200 = To More Specific Class(target class=w297, reference=w275) -> (specific class reference=w296:refnum<vi>)  [unwired: 1 in, 1 out]
            n201 = local write "Xmin"(w284) -> ()
            n202 = local write "Ymin"(w283) -> ()
            n203 = local write "Zmin"(w282) -> ()
            n204 = local write "Xmax"(w281) -> ()
            n205 = local write "Ymax"(w280) -> ()
            n206 = local write "Zmax"(w279) -> ()
            n207 = local write "Xcen"(w278) -> ()
            n208 = local write "Ycen"(w277) -> ()
            n209 = local write "Zcen"(w276) -> ()
            n210 = property class="SceneMesh"(reference=w296) -> ("Color Array"=w295:T24[])  [unwired: 1 in, 2 out]
            n211 = Index Array(array=w295) -> (element=w294:T24)  [unwired: 1 in]
            n212 = call "RGBA2Color.vi"("RGBA"=w294) -> ("Alpha"=w292:dbl, "Color"=w291:u32)  [unwired: 9 in]
            n213 = Bundle(cluster=T5 {"Alpha"=1.0, "Color"=0} ("Color"), "Alpha"=w292, "Color"=w291) -> (w290:T5)
            n214 = local write "Model Color"(w290) -> ()
          }
          event "XLR", "XRR", "YLR", "YRR", "ZLR", "ZRR": Mouse Up {
            n215 = event-data() -> ("CtlRef"=w327:refnum<vi>)  [unwired: 1 in, 7 out]
            n216 = local read "Model Selector"() -> (w328:u16)
            n217 = property on="Model Selector" class="Ring (strict)"() -> ("StringsAndValues[]"=w335:T8)  [unwired: 2 in, 2 out]
            n218 = property class="Bool (strict)"(reference=w327) -> ("Label.Text"=w326:string)  [unwired: 1 in, 2 out]
            n219 = Index Array(array=w335, index=w328) -> (element=w334:cluster{"String":string, "Value":u16})
            n220 = Unbundle By Name(w334) -> ("String"=w333:string)
            n221 = case shown="\"XLR\", Default" w326 {
              tunnel: T15 {"Axis"=enum."X", "Angle"=0.0} ("Rotation") -> [w339 w344 w348 w353 w357 w362]
              tunnel: "XR" -> [w337 w341 _ _ _ _]
              tunnel: [w336 w342 w346 w351 w355 w360] -> w322
              tunnel: "YR" -> [_ _ w345 w350 _ _]
              tunnel: "ZR" -> [_ _ _ _ w354 w359]
              frame "XLR", Default {
                n222 = Bundle By Name(cluster=w339, "Axis"=enum16{"X", "Y", "Z"}."X", "Angle"=w337) -> (w336:T15)
              }
              frame "XRR" {
                n223 = Negate(x=w341) -> (-x=w340:dbl)
                n224 = Bundle By Name(cluster=w344, "Axis"=enum16{"X", "Y", "Z"}."X", "Angle"=w340) -> (w342:T15)
              }
              frame "YLR" {
                n225 = Bundle By Name(cluster=w348, "Axis"=enum16{"X", "Y", "Z"}."Y", "Angle"=w345) -> (w346:T15)
              }
              frame "YRR" {
                n226 = Negate(x=w350) -> (-x=w349:dbl)
                n227 = Bundle By Name(cluster=w353, "Axis"=enum16{"X", "Y", "Z"}."Y", "Angle"=w349) -> (w351:T15)
              }
              frame "ZLR" {
                n228 = Bundle By Name(cluster=w357, "Axis"=enum16{"X", "Y", "Z"}."Z", "Angle"=w354) -> (w355:T15)
              }
              frame "ZRR" {
                n229 = Negate(x=w359) -> (-x=w358:dbl)
                n230 = Bundle By Name(cluster=w362, "Axis"=enum16{"X", "Y", "Z"}."Z", "Angle"=w358) -> (w360:T15)
              }
            }
            n231 = Concatenate Strings("Model" ("string"), w333) -> (w325:string)
            n232 = call "ObjectTable.vi"("ObjectStoreSelector"=T7."Find", "Name"="World") -> ("ObjectRef"=w329:refnum<vi>)  [unwired: 5 in, 4 out]
            n233 = call <vilib>:"Find Object.vi"("Object Name"=w325, "Scene Refnum"=w329) -> ("Object Refnum"=w320:refnum<vi>)  [unwired: 8 in, 1 out]
            n234 = local read "Model Color"() -> (w319:T5)
            n235 = call "TriangleCache.vi"("Rotation"=w322, "TriangleOperations"=T6."Rotate", "ModelName"=w325) -> ("TrianglesOut"=w303:T17[])  [unwired: 8 in]
            n236 = call "Triangle2Mesh.vi"("Color"=w319, "Triangles"=w303) -> ("Refnum"=w318:refnum<vi>)  [unwired: 9 in]
            n237 = invoke class="SceneObject" method="Set Drawable"(reference=w320, "Drawable"=w318) -> ()  [unwired: 2 in, 4 out]
            n238 = call "TrianglesMaxMin.vi"("Triangles"=w303) -> ("Center"=w313:T16, "MaxDims"=w314:T16, "MinDims"=w315:T16)  [unwired: 8 in]
            n239 = Unbundle By Name(w315) -> ("X"=w312:sgl, "Y"=w311:sgl, "Z"=w310:sgl)
            n240 = Unbundle By Name(w314) -> ("X"=w309:sgl, "Y"=w308:sgl, "Z"=w307:sgl)
            n241 = Unbundle By Name(w313) -> ("X"=w306:sgl, "Y"=w305:sgl, "Z"=w304:sgl)
            n242 = local write "Xmin"(w312) -> ()
            n243 = local write "Ymin"(w311) -> ()
            n244 = local write "Zmin"(w310) -> ()
            n245 = local write "Xmax"(w309) -> ()
            n246 = local write "Ymax"(w308) -> ()
            n247 = local write "Zmax"(w307) -> ()
            n248 = local write "Xcen"(w306) -> ()
            n249 = local write "Ycen"(w305) -> ()
            n250 = local write "Zcen"(w304) -> ()
          }
          event "XNT", "YNT", "ZNT", "XPT", "YPT", "ZPT": Mouse Up {
            n251 = event-data() -> ("CtlRef"=w368:refnum<vi>)  [unwired: 1 in, 7 out]
            n252 = local read "Model Selector"() -> (w388:u16)
            n253 = property on="Model Selector" class="Ring (strict)"() -> ("StringsAndValues[]"=w395:T8)  [unwired: 2 in, 2 out]
            n254 = property class="Bool (strict)"(reference=w368) -> ("Label.Text"=w387:string)  [unwired: 1 in, 2 out]
            n255 = Index Array(array=w395, index=w388) -> (element=w394:cluster{"String":string, "Value":u16})
            n256 = Unbundle By Name(w394) -> ("String"=w393:string)
            n257 = case shown="\"XPT\", Default" w387 {
              tunnel: T16 {"X"=0.0, "Y"=0.0, "Z"=0.0} ("Point3D") -> [w398 w402 w405 w409 w412 w416]
              tunnel: "XT" -> [w397 w400 _ _ _ _]
              tunnel: [w396 w401 w404 w408 w411 w415] -> w364
              tunnel: "YT" -> [_ _ w403 w407 _ _]
              tunnel: "ZT" -> [_ _ _ _ w410 w414]
              frame "XPT", Default {
                n258 = Bundle By Name(cluster=w398, "X"=w397) -> (w396:T16)
              }
              frame "XNT" {
                n259 = Negate(x=w400) -> (-x=w399:dbl)
                n260 = Bundle By Name(cluster=w402, "X"=w399) -> (w401:T16)
              }
              frame "YPT" {
                n261 = Bundle By Name(cluster=w405, "Y"=w403) -> (w404:T16)
              }
              frame "YNT" {
                n262 = Negate(x=w407) -> (-x=w406:dbl)
                n263 = Bundle By Name(cluster=w409, "Y"=w406) -> (w408:T16)
              }
              frame "ZPT" {
                n264 = Bundle By Name(cluster=w412, "Z"=w410) -> (w411:T16)
              }
              frame "ZNT" {
                n265 = Negate(x=w414) -> (-x=w413:dbl)
                n266 = Bundle By Name(cluster=w416, "Z"=w413) -> (w415:T16)
              }
            }
            n267 = Concatenate Strings("Model" ("string"), w393) -> (w386:string)
            n268 = call "ObjectTable.vi"("ObjectStoreSelector"=T7."Find", "Name"="World") -> ("ObjectRef"=w389:refnum<vi>)  [unwired: 5 in, 4 out]
            n269 = call <vilib>:"Find Object.vi"("Object Name"=w386, "Scene Refnum"=w389) -> ("Object Refnum"=w384:refnum<vi>)  [unwired: 8 in, 1 out]
            n270 = local read "Model Color"() -> (w383:T5)
            n271 = call "TriangleCache.vi"("Point3D"=w364, "TriangleOperations"=T6."Translate", "ModelName"=w386) -> ("TrianglesOut"=w369:T17[])  [unwired: 8 in]
            n272 = call "Triangle2Mesh.vi"("Color"=w383, "Triangles"=w369) -> ("Refnum"=w382:refnum<vi>)  [unwired: 9 in]
            n273 = invoke class="SceneObject" method="Set Drawable"(reference=w384, "Drawable"=w382) -> ()  [unwired: 2 in, 4 out]
            n274 = call "TrianglesMaxMin.vi"("Triangles"=w369) -> ("Center"=w379:T16, "MaxDims"=w380:T16, "MinDims"=w381:T16)  [unwired: 8 in]
            n275 = Unbundle By Name(w381) -> ("X"=w378:sgl, "Y"=w377:sgl, "Z"=w376:sgl)
            n276 = Unbundle By Name(w380) -> ("X"=w375:sgl, "Y"=w374:sgl, "Z"=w373:sgl)
            n277 = Unbundle By Name(w379) -> ("X"=w372:sgl, "Y"=w371:sgl, "Z"=w370:sgl)
            n278 = local write "Xmin"(w378) -> ()
            n279 = local write "Ymin"(w377) -> ()
            n280 = local write "Zmin"(w376) -> ()
            n281 = local write "Xmax"(w375) -> ()
            n282 = local write "Ymax"(w374) -> ()
            n283 = local write "Zmax"(w373) -> ()
            n284 = local write "Xcen"(w372) -> ()
            n285 = local write "Ycen"(w371) -> ()
            n286 = local write "Zcen"(w370) -> ()
          }
          event "Scale": Mouse Up {
            n287 = event-data() -> ()  [unwired: 1 in, 8 out]
            n288 = local read "Model Selector"() -> (w437:u16)
            n289 = property on="Model Selector" class="Ring (strict)"() -> ("StringsAndValues[]"=w444:T8)  [unwired: 2 in, 2 out]
            n290 = Index Array(array=w444, index=w437) -> (element=w443:cluster{"String":string, "Value":u16})
            n291 = Unbundle By Name(w443) -> ("String"=w442:string)
            n292 = Concatenate Strings("Model" ("string"), w442) -> (w436:string)
            n293 = call "ObjectTable.vi"("ObjectStoreSelector"=T7."Find", "Name"="World") -> ("ObjectRef"=w438:refnum<vi>)  [unwired: 5 in, 4 out]
            n294 = call <vilib>:"Find Object.vi"("Object Name"=w436, "Scene Refnum"=w438) -> ("Object Refnum"=w434:refnum<vi>)  [unwired: 8 in, 1 out]
            n295 = expression code="x/100"("Percent") -> (w417:dbl)
            n296 = local read "Model Color"() -> (w433:T5)
            n297 = call "TriangleCache.vi"("TriangleOperations"=T6."Scale", "ScaleFac"=w417, "ModelName"=w436) -> ("TrianglesOut"=w419:T17[])  [unwired: 8 in]
            n298 = call "Triangle2Mesh.vi"("Color"=w433, "Triangles"=w419) -> ("Refnum"=w432:refnum<vi>)  [unwired: 9 in]
            n299 = invoke class="SceneObject" method="Set Drawable"(reference=w434, "Drawable"=w432) -> ()  [unwired: 2 in, 4 out]
            n300 = call "TrianglesMaxMin.vi"("Triangles"=w419) -> ("Center"=w429:T16, "MaxDims"=w430:T16, "MinDims"=w431:T16)  [unwired: 8 in]
            n301 = Unbundle By Name(w431) -> ("X"=w428:sgl, "Y"=w427:sgl, "Z"=w426:sgl)
            n302 = Unbundle By Name(w430) -> ("X"=w425:sgl, "Y"=w424:sgl, "Z"=w423:sgl)
            n303 = Unbundle By Name(w429) -> ("X"=w422:sgl, "Y"=w421:sgl, "Z"=w420:sgl)
            n304 = local write "Xmin"(w428) -> ()
            n305 = local write "Ymin"(w427) -> ()
            n306 = local write "Zmin"(w426) -> ()
            n307 = local write "Xmax"(w425) -> ()
            n308 = local write "Ymax"(w424) -> ()
            n309 = local write "Zmax"(w423) -> ()
            n310 = local write "Xcen"(w422) -> ()
            n311 = local write "Ycen"(w421) -> ()
            n312 = local write "Zcen"(w420) -> ()
          }
          event Value Change {
            n313 = event-data() -> ("NewVal"=w445:T5)  [unwired: 1 in, 5 out]
            n314 = local read "Model Selector"() -> (w451:u16)
            n315 = property on="Model Selector" class="Ring (strict)"() -> ("StringsAndValues[]"=w458:T8)  [unwired: 2 in, 2 out]
            n316 = Index Array(array=w458, index=w451) -> (element=w457:cluster{"String":string, "Value":u16})
            n317 = Unbundle By Name(w457) -> ("String"=w456:string)
            n318 = Concatenate Strings("Model" ("string"), w456) -> (w450:string)
            n319 = call "ObjectTable.vi"("ObjectStoreSelector"=T7."Find", "Name"="World") -> ("ObjectRef"=w452:refnum<vi>)  [unwired: 5 in, 4 out]
            n320 = call <vilib>:"Find Object.vi"("Object Name"=w450, "Scene Refnum"=w452) -> ("Object Refnum"=w448:refnum<vi>)  [unwired: 8 in, 1 out]
            n321 = call "TriangleCache.vi"("TriangleOperations"=T6."Get", "ModelName"=w450) -> ("TrianglesOut"=w446:T17[])  [unwired: 9 in]
            n322 = call "Triangle2Mesh.vi"("Color"=w445, "Triangles"=w446) -> ("Refnum"=w447:refnum<vi>)  [unwired: 9 in]
            n323 = invoke class="SceneObject" method="Set Drawable"(reference=w448, "Drawable"=w447) -> ()  [unwired: 2 in, 4 out]
          }
          event "SaveSCAN": Mouse Up {
            n324 = event-data() -> ()  [unwired: 1 in, 8 out]
            n325 = call "File Dialog4"("prompt"="Choose location to save SCAN...", "default name"="SCAN.xml", "pattern (all files)"="*.xml", "pattern label"="XML") -> ("selected path"=w459:path, "cancelled"=w460:bool)  [unwired: 8 in, 2 out]
            n326 = case shown="False" w460 {
              tunnel: w459 -> [w466 _]
              frame False {
                n327 = local read "SCAN"() -> (w467:T1)
                n328 = Flatten To XML(anything=w467) -> (xml string=w465:string)
                n329 = Write to Text File(file (use dialog)=w466, text=w465) -> ()  [unwired: 2 in, 3 out]
              }
              frame True {
              }
            }
          }
        }
      }
    }
  }
